vi "Configure Measurement (Time Interval).vi"(8 "error in (no error)":errorcluster, 10 "Measurement Channels (0: Channel1, Channel2)":i32(ring) items=["Channel1, Channel2", "Channel2, Channel1", " Channel1", "Channel2"], 11 "VISA resource name":refnum<visa-resource-name>) -> (0 "error out":errorcluster, 3 "VISA resource name out":refnum<visa-resource-name>)   [LabVIEW 2024, in "Agilent 532XX Series.lvlib"]
doc: "Sets all measurement parameters and trigger parameters to default values for time interval measurements on one channel or between two channels.\n\n<B>Note:</B> This VI only applies to the Agilent 53220A/53230A."
uses:
  Agilent 532XX Series.lvlib
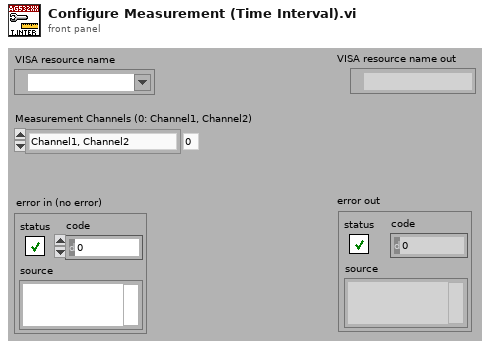
[diagram p1: front panel]
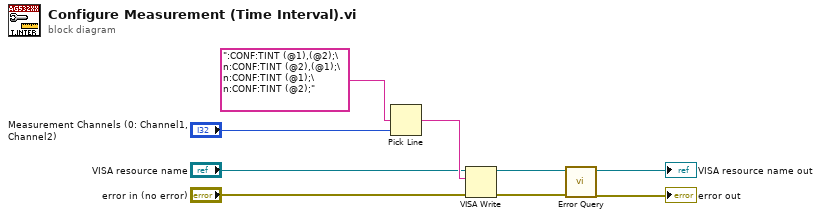
[diagram p0: block diagram]
diagram:
  n1 = Pick Line(multi-line string=":CONF:TINT (@1),(@2);\n:CONF:TINT (@2),(@1);\n:CONF:TINT (@1);\n:CONF:TINT (@2);", line index="Measurement Channels (0: Channel1, Channel2)") -> (output string=w7:string)  [unwired: 1 out]
  n2 = VISA Write(VISA resource name="VISA resource name", write buffer=w7, error in (no error)="error in (no error)") -> (VISA resource name out=w4:refnum<visa-resource-name>, error out=w3:errorcluster)  [unwired: 1 out]
  n3 = call "Error Query.vi"("error in (no error)"=w3, "VISA resource name"=w4) -> ("error out"=→"error out":errorcluster, "VISA resource name out"=→"VISA resource name out":refnum<visa-resource-name>)  [unwired: 8 out]
